vi "Heat2D_X RHS F.vi"(6 "Coefficients":T1, 10 "step":i32, 11 "F(n+1)+F(n)":dbl[][][](array[numeric])) -> (3 "F":dbl[][](array[numeric]))   [LabVIEW 2020, in "NI_PDE.lvlib"]
uses:
  <vilib>/gmath/NI_PDE.lvlib
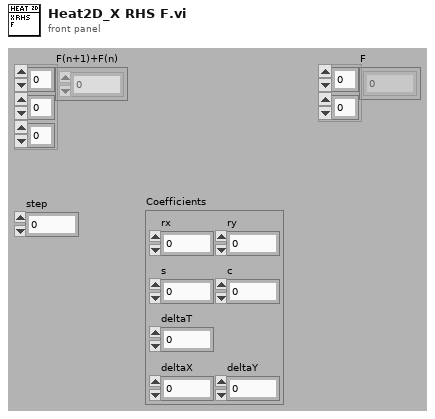
[diagram p1: front panel]
types:
  T1 = cluster{"rx":dbl, "ry":dbl, "s":dbl, "c":dbl, "deltaT":dbl, "deltaX":dbl, "deltaY":dbl}
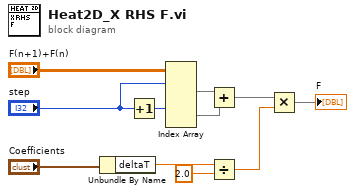
[diagram p0: block diagram]
diagram:
  n1 = Unbundle By Name("Coefficients") -> ("deltaT"=w10:dbl)
  n2 = Increment(x="step") -> (x+1=w7:i32)
  n3 = Index Array(array="F(n+1)+F(n)", index (dim 0) #1="step", index (dim 0) #2=w7) -> (element #1=w5:dbl[][], element #2=w6:dbl[][])  [unwired: 4 in]
  n4 = Add(x=w5, y=w6) -> (x+y=w2:dbl[][])
  n5 = Divide(x=w10, y=2.0 ("value")) -> (x/y=w9:dbl)
  n6 = Multiply(x=w2, y=w9) -> (x*y=→"F":dbl[][])
